vi "Extract Fill Stroke From Style.vi"(0 "Array of Results":string[](array[string])) -> (1 "Fill":string, 2 "Stroke":string)   [LabVIEW 2019]
doc: "This VI gets fill and stroke color from the array of XPath results for style."
uses:
  <vilib>/regexp/Match Regular Expression.xnode
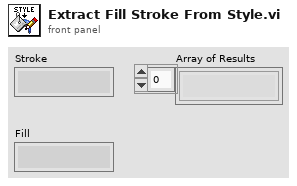
[diagram p1: front panel]
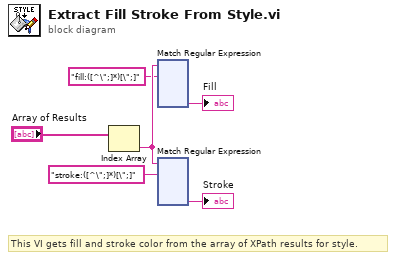
[diagram p0: block diagram]
diagram:
  # "This VI gets fill and stroke color from the array of XPath results for style."
  n1 = Index Array(array="Array of Results") -> (element=w4:string)  [unwired: 1 in]
  n2 = xnode "Match Regular Expression"("input string"=w4, "regular expression"="fill:([^\";]*)[\";]") -> ("submatch 1"=→"Fill":string)  [unwired: 4 in, 5 out]
  n3 = xnode "Match Regular Expression"("input string"=w4, "regular expression"="stroke:([^\";]*)[\";]") -> ("submatch 1"=→"Stroke":string)  [unwired: 4 in, 5 out]
